vi "Set DataCell (String).vi"(0 "DataGridView in":refnum<class "DataGridView.lvclass">, 5 "row index":i32, 7 "col index":i32, 9 "Data":string, 11 "error in":errorcluster) -> (4 "DataGridView out":refnum<class "DataGridView.lvclass">, 15 "error out":errorcluster)   [LabVIEW 2016, in "DataGrid.lvlib" / "DataGridView.lvclass"]
uses:
  <userlib>/LabVIEWdotNetDataGrid/source/DataGridView/DataGridView.lvclass
  <userlib>/LabVIEWdotNetDataGrid/source/DataGridView/DataGridView.lvclass/DataGridView.ctl
  System.Windows.Forms
  <userlib>/LabVIEWdotNetDataGrid/source/DataTable/DataTable.lvclass
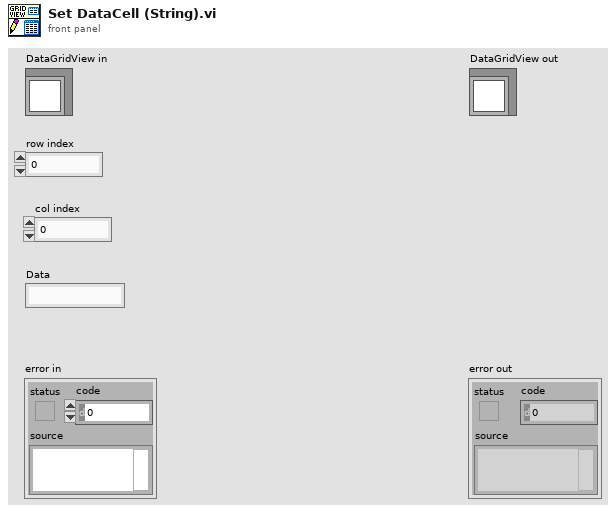
[diagram p1: front panel]
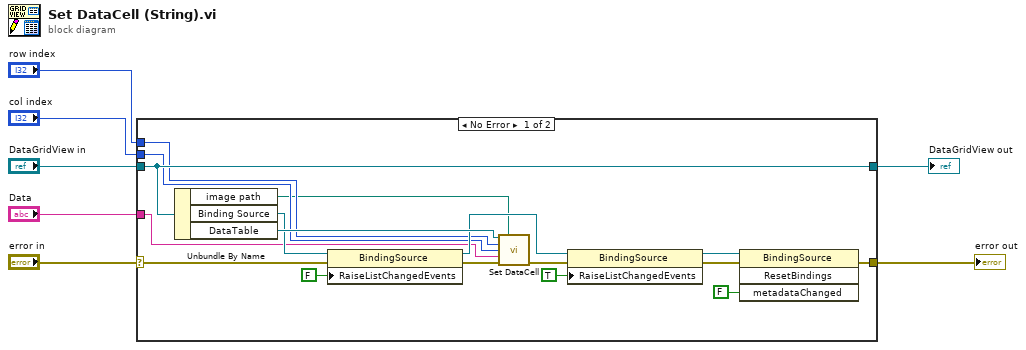
[diagram p0: block diagram]
diagram:
  n1 = case shown="No Error" "error in" {
    selector: "error in" -> [w20 w25]
    tunnel: [w17 w25] -> w6
    tunnel: [w24 w26] -> w4
    tunnel: "DataGridView in" -> [w24 w26]
    tunnel: "Data" -> [w11 _]
    tunnel: "col index" -> [w10 _]
    tunnel: "row index" -> [w9 _]
    frame No Error {
      n2 = Unbundle By Name(w24) -> ("image path"=w8:path, "Binding Source"=w22:refnum<k24>, "DataTable"=w23:refnum<class "DataTable.lvclass">)
      n3 = property class="BindingSource"(reference=w22, error in=w20, "RaiseListChangedEvents"=FALSE) -> (reference out=w21:refnum<k24>, error out=w19:errorcluster)
      n4 = call-poly <userlib>:"Set DataCell.vi"("DataTable in"=w23, "image path"=w8, "row index"=w9, "col index"=w10, "String Data"=w11, "error in (no error)"=w19) -> ("error out"=w18:errorcluster)  [unwired: 8 in, 1 out]
      n5 = property class="BindingSource"(reference=w21, error in=w18, "RaiseListChangedEvents"=TRUE) -> (reference out=w14:refnum<k24>, error out=w15:errorcluster)
      n6 = invoke class="BindingSource" method="ResetBindings"(reference=w14, error in=w15, "metadataChanged"=FALSE) -> (error out=w17:errorcluster)  [unwired: 1 in, 3 out]
    }
    frame Error {
    }
  }
  "error out" <- w6
  "DataGridView out" <- w4
